vi "Initialize Lookup Table -Triangle.vi"() -> ()   [LabVIEW 2015]
uses:
  <vilib>/measure/NI_MABase.lvlib
panel:
  out "波形图":i16[](graph)
  out "Init Data Out":i16[](array[numeric])
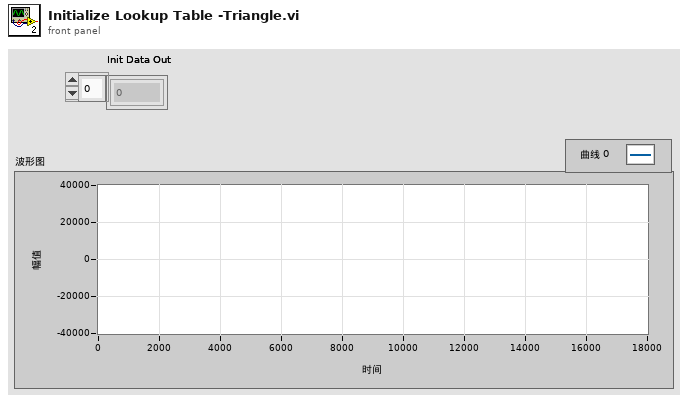
[diagram p1: front panel]
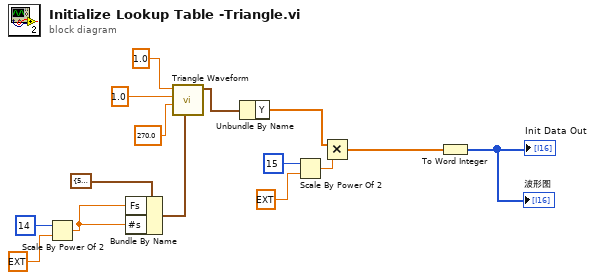
[diagram p0: block diagram]
diagram:
  n1 = Scale By Power Of 2(n=i16 14, x=ext 1.0) -> (x*2^n=w12:ext)
  n2 = Bundle By Name(cluster=cluster{"Fs":dbl, "#s":dbl} {"Fs"=5000.0, "#s"=50.0} ("sampling info"), "Fs"=w12, "#s"=w12) -> (w4:cluster{"Fs":dbl, "#s":dbl})
  n3 = call <vilib>:"Triangle Waveform.vi"("sampling info"=w4, "phase"=270.0, "amplitude"=1.0, "frequency"=1.0) -> ("signal out"=w7:waveform(dbl))  [unwired: 6 in, 1 out]
  n4 = Unbundle By Name(w7) -> ("Y"=w5:dbl[])
  n5 = Scale By Power Of 2(n=i16 15, x=ext 1.0) -> (x*2^n=w9:ext)
  n6 = Multiply(x=w5, y=w9) -> (x*y=w6:ext[])
  n7 = To Word Integer(number=w6) -> (16bit integer=→"Init Data Out" →"波形图":i16[])
